vi "BRig_comm_webdav_myrioPassword.vi"() -> (2 "output_myrioPassword":string)   [LabVIEW 2014]
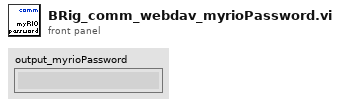
[diagram p1: front panel]
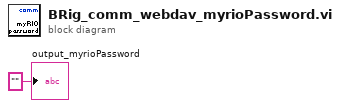
[diagram p0: block diagram]
diagram:
  "output_myrioPassword" <- "" ("host uri prefix")
